vi "DAQNavi Read (Counter Count Value 1Chan 1Samp).vi"(8 "error in (no error)":errorcluster, 10 "timeout":dbl=10.0, 11 "task in":i32) -> (0 "error out":errorcluster, 2 "data":i32, 3 "task out":i32)   [LabVIEW 2020]
uses:
  DAQNavi_LV.dll
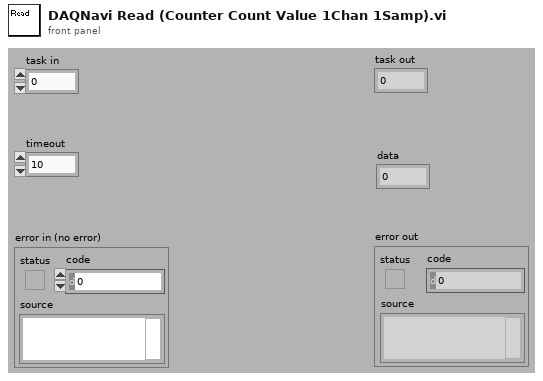
[diagram p1: front panel]
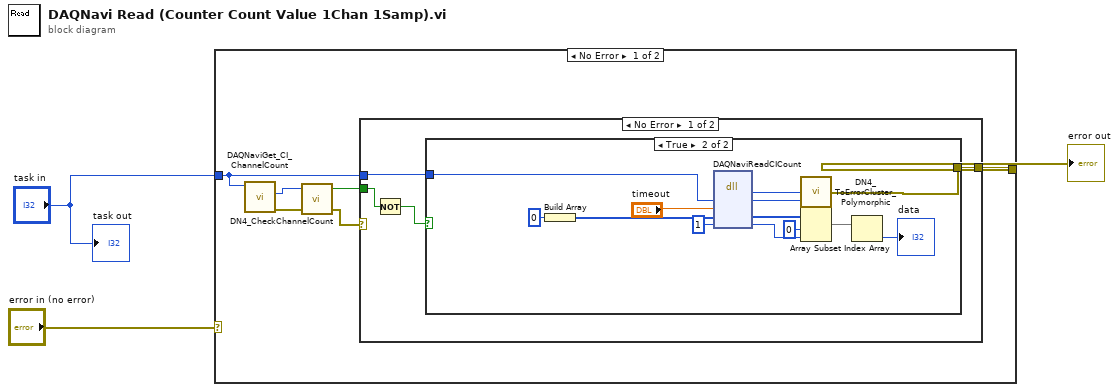
[diagram p0: block diagram]
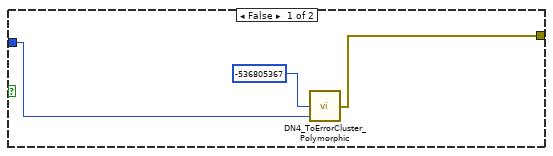
[diagram p2: hidden frame]
diagram:
  n1 = case shown="No Error" "error in (no error)" {
    selector: "error in (no error)" -> [_ w31]
    tunnel: "task in" -> [w8 _]
    tunnel: [w9 w31] -> w1
    frame No Error {
      n2 = call "DAQNaviGet_CI_ChannelCount.vi"("task in"=w8) -> ("error out"=w7:errorcluster, "channel count"=w6:i32)  [unwired: 1 in, 8 out]
      n3 = call "DN4_CheckChannelCount.vi"("error out"=w7, "channel count"=w6) -> ("error IO"=w5:errorcluster, "greater than 1?"=w4:bool)  [unwired: 2 out]
      n4 = case shown="No Error" w5 {
        selector: w5 -> [_ w30]
        tunnel: [w13 w30] -> w9
        tunnel: w8 -> [w12 _]
        tunnel: w4 -> [w10 _]
        frame No Error {
          n5 = Not(x=w10) -> (.not. x?=w11:bool)
          n6 = case shown="True" w11 {
            tunnel: [w14 w29] -> w13
            tunnel: w12 -> [w15 w17]
            frame False {
              n7 = call "DN4_ToErrorCluster_Polymorphic.vi"("task id"=w15, "error code"=-536805367) -> ("error out"=w14:errorcluster)  [unwired: 3 out]
            }
            frame True {
              n8 = Build Array(0 ("element")) -> (w25:i32[])
              n9 = dll-call lib="DAQNavi_LV.dll" fn="DAQNaviReadCICount"("taskID"=w17, "timeout"="timeout", "count"=w25, "samples"=u32 1) -> ("return type"=w28:i32, "taskID"=w18:i32, "count"=w24:i32[], "samples"=w22:u32)  [unwired: 4 in, 2 out]
              n10 = call "DN4_ToErrorCluster_Polymorphic.vi"("task id"=w18, "error code"=w28) -> ("error out"=w29:errorcluster)  [unwired: 3 out]
              n11 = Array Subset(array=w24, index=0, length=w22) -> (w20:i32[])
              n12 = Index Array(array=w20) -> (element=→"data":i32)  [unwired: 1 in]
            }
          }
        }
        frame Error {
        }
      }
    }
    frame Error {
    }
  }
  "error out" <- w1
  "task out" <- "task in"
